vi "list_img.vi"(8 "error in":errorcluster, 11 "Input path":path) -> (0 "error out":errorcluster, 3 "Output list of paths":path[](array[path]))   [LabVIEW 2020]
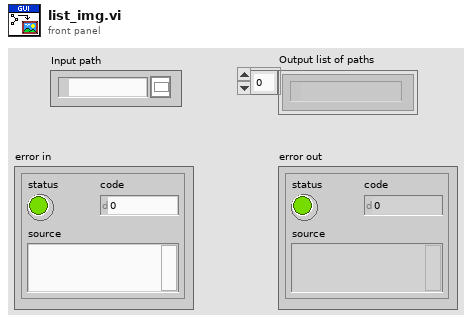
[diagram p1: front panel]
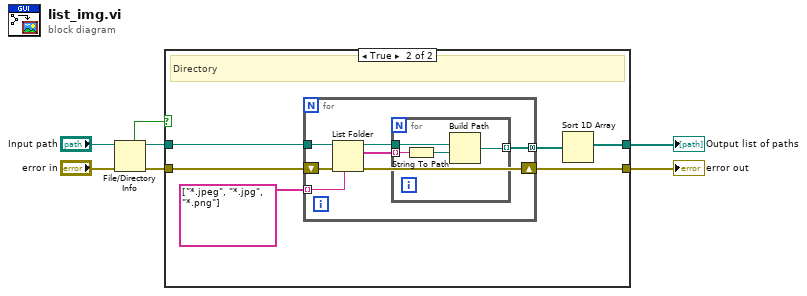
[diagram p0: block diagram]
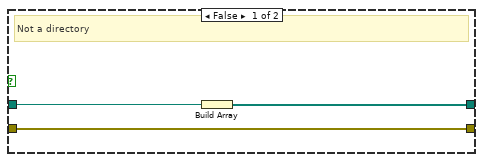
[diagram p2: hidden frame]
diagram:
  n1 = File/Directory Info(path="Input path", error in="error in") -> (path out=w7:path, directory=w6:bool, error out=w5:errorcluster)  [unwired: 4 out]
  n2 = case shown="True" w6 {
    tunnel: w5 -> [w10 w16]
    tunnel: [w10 w15] -> w1
    tunnel: w7 -> [w9 w13]
    tunnel: [w8 w11] -> w3
    frame False {
      # "Not a directory"
      n3 = Build Array(w9) -> (w8:path[])
    }
    frame True {
      # "Directory"
      n4 = for {
        tunnel: w13 -> [w20]
        tunnel: string[] ["*.jpeg", "*.jpg", "*.png"] ("pattern") -> [w21] mode=indexing
        shift-right: [w22] -> w15
        shift-left: w16 -> [w23]
        tunnel: [w19] -> w12 mode=concatenating
        n5 = List Folder(path=w20, pattern=w21, error in=w23) -> (path out=w18:path, filenames=w17:string[], error out=w22:errorcluster)  [unwired: 1 in, 1 out]
        n6 = for {
          tunnel: w18 -> [w26]
          tunnel: w17 -> [w27] mode=indexing
          tunnel: [w24] -> w19 mode=indexing
          n7 = String To Path(string=w27) -> (path=w25:path)
          n8 = Build Path(base path=w26, name or relative path=w25) -> (appended path=w24:path)
        }
      }
      n9 = Sort 1D Array(array=w12) -> (sorted array=w11:path[])
    }
  }
  "error out" <- w1
  "Output list of paths" <- w3
